vi "CM-Change Breakout Box Type.vi"(0 "slot ctl refs":refnum<vi>[](array[refnum]), 5 "Devices":T1[](array[typedef]), 9 "Breakout box type":enum32{"BNC-2090", "BNC-2110"}(radio), 11 "error in (no error)":errorcluster) -> (15 "error out":errorcluster)   [LabVIEW 2015]
uses:
  Type Defs/General PXISlot XControl/PXISlotGP.xctl
  PXI DAQ VIs/Type Defs/PXI-Device Spec.ctl
  Type Defs/PXISlot XControl/Connector Type.ctl
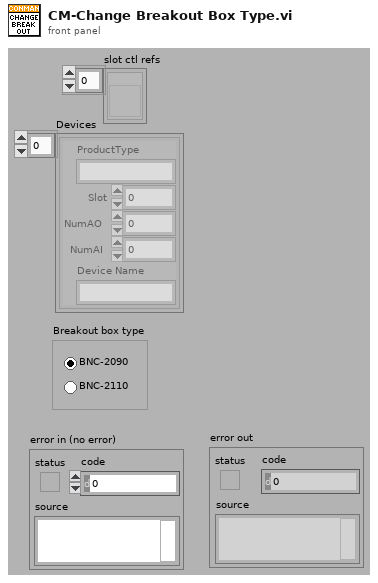
[diagram p1: front panel]
types:
  T1 = typedef "PXI-Device Spec.ctl" = cluster{"Slot":i32, "ProductType":string, "NumAO":i32, "NumAI":i32, "Device Name":string}
  T2 = typedef "Connector Type.ctl" = enum16{"None", "PXI-4461", "BNC-2110", "BNC-2090"}
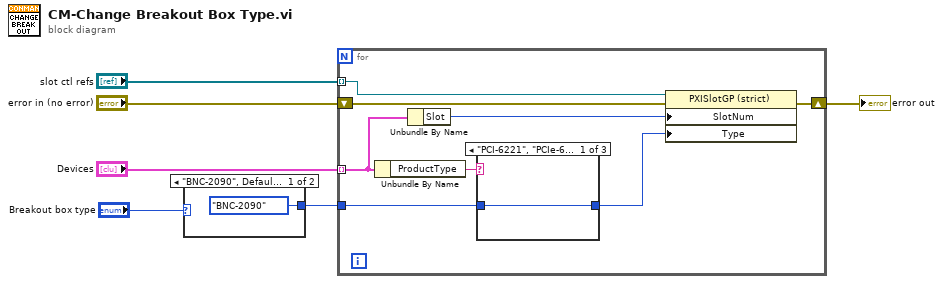
[diagram p0: block diagram]
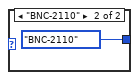
[diagram p2: hidden frame]
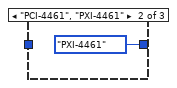
[diagram p3: hidden frame]
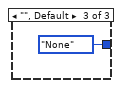
[diagram p4: hidden frame]
diagram:
  n1 = case shown="\"BNC-2090\", Default" "Breakout box type" {
    tunnel: [Connector_Type."BNC-2090" ("Connector Type") Connector_Type."BNC-2110" ("Connector Type")] -> w1
    frame "BNC-2090", Default {
    }
    frame "BNC-2110" {
    }
  }
  n2 = for {
    tunnel: "slot ctl refs" -> [w9] mode=indexing
    shift-right: [w15] -> w5
    shift-left: "error in (no error)" -> [w16]
    tunnel: "Devices" -> [w11] mode=indexing
    tunnel: w1 -> [w13]
    n3 = Unbundle By Name(w11) -> ("ProductType"=w14:string)
    n4 = Unbundle By Name(w11) -> ("Slot"=w10:i32)
    n5 = case shown="\"PCI-6221\", \"PCIe-6321\", \"PXI-6221\", \"PXIe-6341\", \"USB-6002\", \"USB-6221 (BNC)\", \"USB-6341 (BNC)\"" w14 {
      tunnel: w13 -> [w17 _ _]
      tunnel: [w17 Connector_Type."PXI-4461" ("Connector Type") Connector_Type."None" ("Connector Type")] -> w12
      frame "PCI-6221", "PCIe-6321", "PXI-6221", "PXIe-6341", "USB-6002", "USB-6221 (BNC)", "USB-6341 (BNC)" {
      }
      frame "PCI-4461", "PXI-4461" {
      }
      frame "", Default {
      }
    }
    n6 = property class="PXISlotGP (strict)"(reference=w9, error in=w16, "SlotNum"=w10, "Type"=w12) -> (error out=w15:errorcluster)  [unwired: 1 out]
  }
  "error out" <- w5
